vi "Enabled Bool to Disabled Enum.vi"(1 "Enabled?":bool) -> (0 "Disabled":T1(ring))   [LabVIEW 2014, in "COSYLib.lvlib"]
doc: "Converts a boolean describing whether a control should be enabled, to a \"Disabled\" state suitable for wiring to the \"Disabled\" property of a LV control.\nNote that 'disabled' corresponds to \"Disabled & Grayed Out\"."
uses:
  COSYLib.lvlib
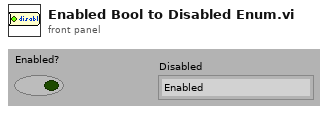
[diagram p1: front panel]
types:
  T1 = enum8{"Enabled", "Disabled", "Disabled and Grayed Out"}
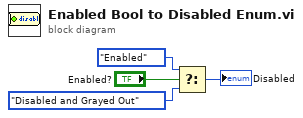
[diagram p0: block diagram]
diagram:
  n1 = Select(t=T1."Enabled" ("Disabled"), s="Enabled?", f=T1."Disabled and Grayed Out") -> (s? t:f=→"Disabled":T1)
